vi "ReadConfig.vi"(0 "reference in":refnum<class "NeedleValve.lvclass">, 11 "error in (no error)":errorcluster) -> (4 "reference out":refnum<class "NeedleValve.lvclass">, 15 "error out":errorcluster)   [LabVIEW 2019, in "NeedleValve.lvclass"]
uses:
  NeedleValve.lvclass
  D:/GIT H4000/H4000/src/Device_class/Device.lvclass
  D:/GIT H4000/H4000/src/Proccess_class/Proccess.lvclass
  Proccess_class/Proccess.lvclass/Proccess.ctl
  Device_class/Device.lvclass/Device.ctl
  NeedleValve.lvclass/NeedleValve.ctl
  32b4956d-1d2c-430c-854c-873c41fce1cb.vi
  <vilib>/Utility/error.llb/Clear Errors.vi
  ConfigInterface_class/ConfigInterface.lvclass
  Proccess_class/Proccess.lvclass
  Device_class/Device.lvclass
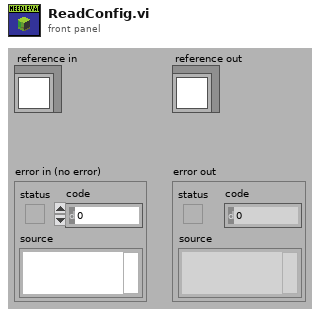
[diagram p1: front panel]
types:
  T1 = typedef "Needle Valve Settings.ctl" = cluster{"average size":i32, "open force":u16, "close force":u16, "open settings":T2, "close settings":T2, "Offset angle":dbl, "Start angle":dbl}
  T2 = typedef "MB_ENGINE.lvclass/Settings.ctl" = cluster{"ACC Steps Per Sec^2":u16, "DEC Steps Per Sec^2":u16, "Min Velosity Step Per Sec":u16, "Max Velosity Step Per Sec":u16, "MicroStep":u16}
  T3 = typedef "Proccess.lvclass/TAGs.ctl" = cluster{"TAG":string, "PTAG":string, "DESC":string}
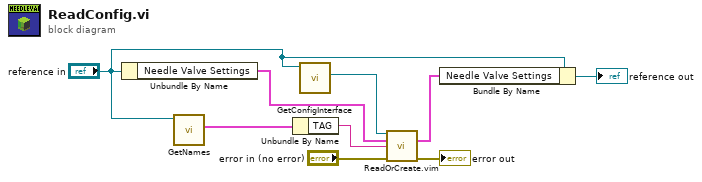
[diagram p0: block diagram]
diagram:
  n1 = Unbundle By Name("reference in") -> ("Needle Valve Settings"=w8:T1)
  n2 = call "GetNames.vi"("Proccess in"="reference in") -> ("Tags"=w6:T3)  [unwired: 10 in]
  n3 = Unbundle By Name(w6) -> ("TAG"=w1:string)
  n4 = call "GetConfigInterface.vi"("Device in"="reference in") -> ("ConfigInterface"=w9:refnum<class "ConfigInterface.lvclass">)  [unwired: 10 in]
  n5 = call "ReadOrCreate.vim"("reference in"=w9, "Type and Defaults"=w8, "Name"=w1, "error in (no error)"="error in (no error)") -> ("Data"=w3:T1, "error out"=→"error out":errorcluster)  [unwired: 7 in, 3 out]
  n6 = Bundle By Name(cluster="reference in", "Needle Valve Settings"=w3) -> (→"reference out":refnum<class "NeedleValve.lvclass">)
